vi "Subvi sample and hold.vi"(7 "Clock":bool, 9 "Input":bool) -> (1 "Output":bool)   [LabVIEW 2017]
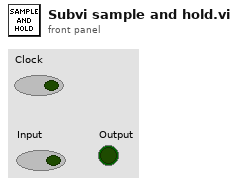
[diagram p1: front panel]
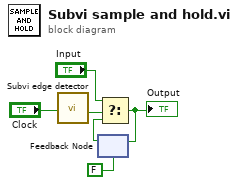
[diagram p0: block diagram]
diagram:
  n1 = call "Subvi edge detector.vi"("Input"="Clock") -> ("Output"=w5:bool)  [unwired: 8 in]
  n2 = feedback #1(FALSE) -> (w2:bool)
  n3 = Select(t="Input", s=w5, f=w2) -> (s? t:f=w1:bool)
  "Output" <- w1
  n4 = feedback-in #1(w1) -> ()
